vi "Shutdown.vi"(8 "error in (no error)":errorcluster) -> (0 "error out":errorcluster)   [LabVIEW 2014]
uses:
  Globals.vi
  <vilib>/vision/driver/NI_Vision_Acquisition_Software.lvlib
  <vilib>/LabVIEW Hacker/LINX/LVH-LINX.lvlib
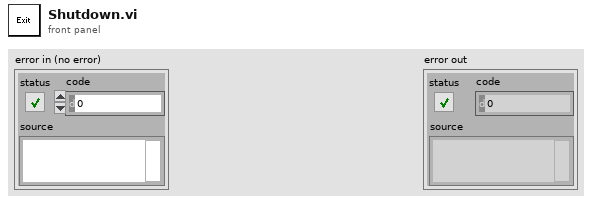
[diagram p1: front panel]
types:
  T1 = typedef "IMAQdx.ctl" = refnum<k21>
  T2 = typedef "LVH-LINX.lvlib/LINX Ref.ctl" = cluster{"Platform":T3, "Interface":T4, "LINX Device Config":T5}
  T3 = typedef "LVH-LINX.lvlib/Platform.ctl" = enum16{"LINX", "myRIO"}
  T4 = typedef "LVH-LINX.lvlib/Interface.ctl" = enum16{"Serial", "TCP"}
  T5 = typedef "LVH-LINX.lvlib/Device.lvlib/LINX Device Config.ctl" = cluster{"Interface":T4, "COM Port":refnum<visa-resource-name>, "TCP Configuration":T6, "Device Family":T7, "Device ID":u8, "Device Name":string, "TCP Ref":refnum<k5>}
  T6 = typedef "LVH-LINX.lvlib/Device.lvlib/TCP Config.ctl" = cluster{"IP Address":string, "Port":u16}
  T7 = typedef "LVH-LINX.lvlib/Device Family.ctl" = enum8{"National Instruments", "Digilent", "Arduino"}
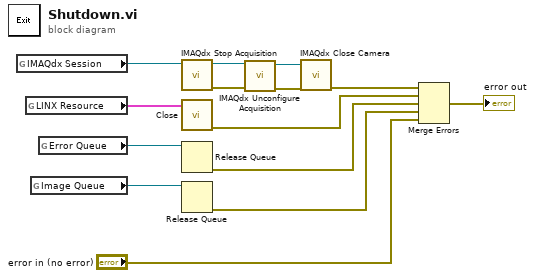
[diagram p0: block diagram]
diagram:
  n1 = global read "Globals.vi" "IMAQdx Session"() -> (w9:T1)
  n2 = global read "Globals.vi" "LINX Resource"() -> (w10:T2)
  n3 = global read "Globals.vi" "Image Queue"() -> (w7:refnum<queue>)
  n4 = global read "Globals.vi" "Error Queue"() -> (w8:refnum<queue>)
  n5 = call <vilib>:"IMAQdx Stop Acquisition.vi"("Session In"=w9) -> ("error out"=w11:errorcluster, "Session Out"=w14:T1)  [unwired: 9 in]
  n6 = call <vilib>:"Close.vi"("LINX Resource"=w10) -> ("Error Out"=w5:errorcluster)  [unwired: 9 in, 1 out]
  n7 = Release Queue(queue=w8) -> (error out=w4:errorcluster)  [unwired: 2 in, 2 out]
  n8 = Release Queue(queue=w7) -> (error out=w3:errorcluster)  [unwired: 2 in, 2 out]
  n9 = call <vilib>:"IMAQdx Unconfigure Acquisition.vi"("error in"=w11, "Session In"=w14) -> ("error out"=w12:errorcluster, "Session Out"=w13:T1)  [unwired: 8 in]
  n10 = call <vilib>:"IMAQdx Close Camera.vi"("error in"=w12, "Session In"=w13) -> ("error out"=w6:errorcluster)  [unwired: 9 in]
  n11 = Merge Errors(w6, w5, w4, w3, "error in (no error)") -> (→"error out":errorcluster)
